vi "Set Buffer and Get Channel Reading.vi"(8 "error in":errorcluster, 9 "Readings":dbl[][](array[numeric]), 10 "Channel Ident":string, 11 "BufferLastReadingsDBL in":refnum<class "BufferLastReadsDBL.lvclass">) -> (0 "error out":errorcluster, 2 "Reading":dbl, 3 "BufferLastReadingsDBL out":refnum<class "BufferLastReadsDBL.lvclass">)   [LabVIEW 2024, in "BufferLastReadsDBL.lvclass"]
uses:
  BufferLastReadsDBL.lvclass
  BufferLastReadsDBL.lvclass/BufferLastReadsDBL.ctl
  <vilib>/Analysis/baseanly.llb/Mean (DBL).vi
  <vilib>/Analysis/NI_AALBase.lvlib
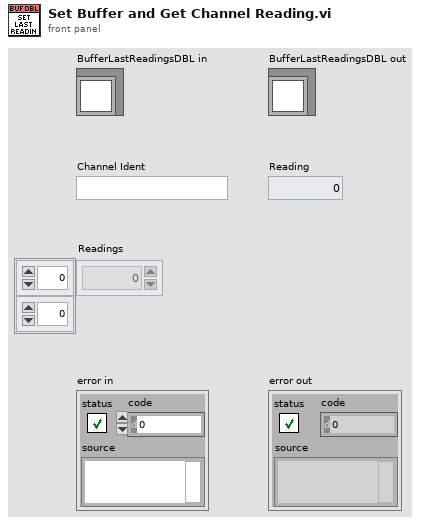
[diagram p1: front panel]
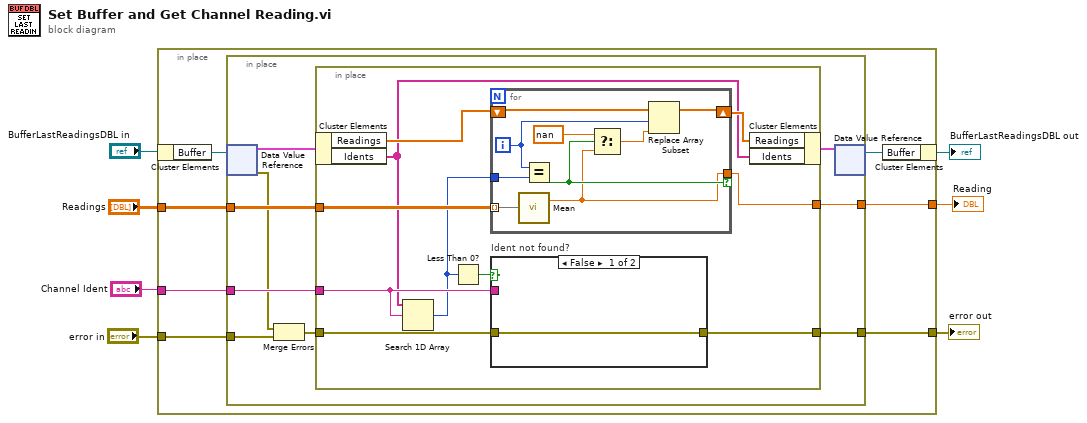
[diagram p0: block diagram]
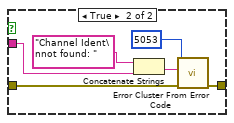
[diagram p2: hidden frame]
diagram:
  n1 = in-place {
    in-place-border: "Readings" -> [w13]
    in-place-border: "error in" -> [w12]
    in-place-border: "Channel Ident" -> [w10]
    in-place-border: [w9] -> w2
    in-place-border: [w8] -> w1
    n2 = in-place-cluster #1("BufferLastReadingsDBL in") -> ("Buffer"=w14:refnum<data-value>)
    n3 = in-place {
      in-place-border: w13 -> [w23]
      in-place-border: w12 -> [w20]
      in-place-border: w10 -> [w22]
      in-place-border: [w17] -> w9
      in-place-border: [w15] -> w8
      n4 = in-place-dvr #2(w14) -> (w18:cluster{"Idents":string[], "Readings":dbl[]}, w19:errorcluster)
      n5 = Merge Errors(w19, w20) -> (w21:errorcluster)
      n6 = in-place {
        in-place-border: w23 -> [w30]
        in-place-border: w22 -> [w32]
        in-place-border: w21 -> [w31]
        in-place-border: [w26] -> w17
        in-place-border: [w25] -> w15
        n7 = in-place-cluster #3(w18) -> ("Readings"=w29:dbl[], "Idents"=w24:string[])
        n8 = Search 1D Array(1D array=w24, element=w32) -> (index of element=w27:i32)  [unwired: 1 in]
        n9 = Less Than 0?(x=w27) -> (x < 0?=w33:bool)
        n10 = for {
          tunnel: [w48] -> w26 if=w49
          tunnel: w30 -> [w46] mode=indexing
          shift-right: [w42] -> w28
          shift-left: w29 -> [w45]
          tunnel: w27 -> [w41]
          i -> [w44]
          n11 = call-poly <vilib>:"Mean.vi"("X"=w46) -> ("mean"=w48:dbl)  [unwired: 1 out]
          n12 = Equal?(x=w44, y=w41) -> (x = y?=w49:bool)
          n13 = Select(t=nan, s=w49, f=w48) -> (s? t:f=w43:dbl)
          n14 = Replace Array Subset(array=w45, new element=w43, index=w44) -> (w42:dbl[])
        }
        n15 = case "Ident not found?" shown="False" w33 {
          tunnel: w31 -> [w34 w40]
          tunnel: w32 -> [_ w36]
          tunnel: [w34 w35] -> w25
          frame False {
          }
          frame True {
            n16 = Concatenate Strings("Channel Ident\nnot found: " ("error message (\"\")"), w36) -> (w37:string)
            n17 = call <vilib>:"Error Cluster From Error Code.vi"("error in (no error)"=w40, "error message (\"\")"=w37, "error code (0)"=5053) -> ("error out"=w35:errorcluster)  [unwired: 6 in]
          }
        }
        n18 = in-place-cluster #3("Readings"=w28, "Idents"=w24) -> (w16:cluster{"Idents":string[], "Readings":dbl[]})
      }
      n19 = in-place-dvr #2(w16) -> (w11:refnum<data-value>)  [unwired: 1 out]
    }
    n20 = in-place-cluster #1("Buffer"=w11) -> (→"BufferLastReadingsDBL out":refnum<class "BufferLastReadsDBL.lvclass">)
  }
  "error out" <- w1
  "Reading" <- w2
